vi "Deep Thought.vi"(8 "Error In":errorcluster) -> (0 "Error Out":errorcluster)   [LabVIEW 2019, in "Deep Thought.lvlib"]
doc: "Simple string based state machine."
uses:
  Deep Thought.lvlib
  <vilib>/ErrorRing/Error Ring.xnode
  Communication/Queues/MHL/MHL.lvlib
  Communication/Notifiers/Sequencer/Sequencer Handshake.lvlib
  <vilib>/Utility/error.llb/Error Cluster From Error Code.vi
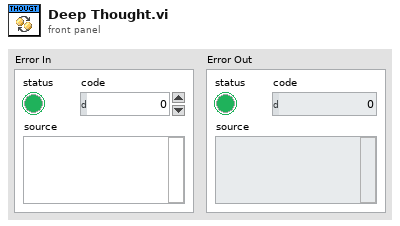
[diagram p1: front panel]
types:
  T1 = enum16{"Obtain", "Send", "Get Notifier", "Release"}
  T2 = enum16{"Obtain", "Enqueue", "Get Queue", "Flush", "Release"}
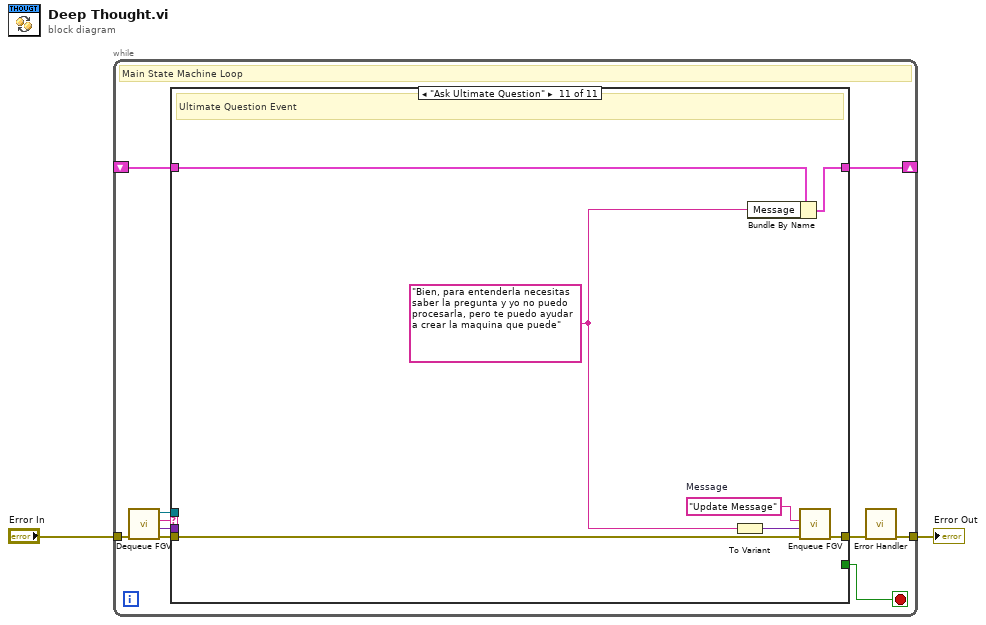
[diagram p0: block diagram]
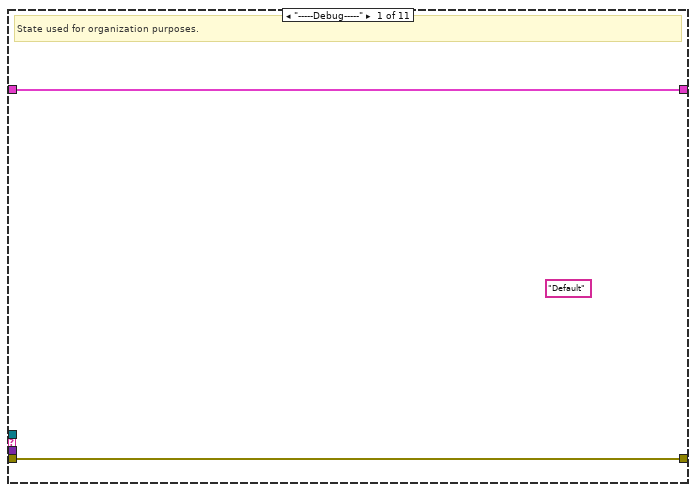
[diagram p2: hidden frame]
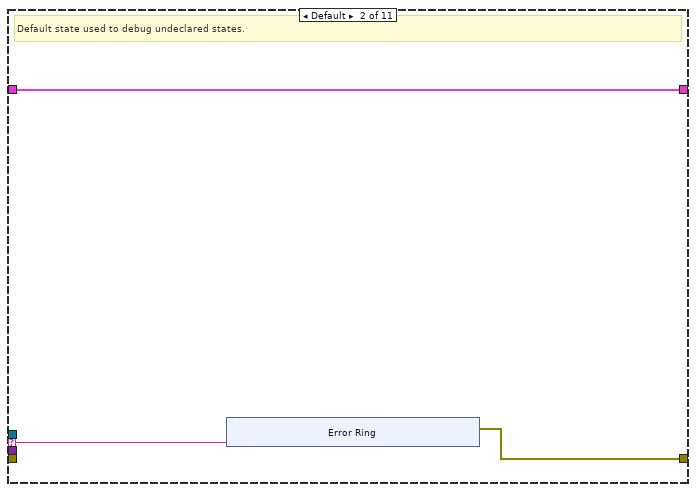
[diagram p3: hidden frame]
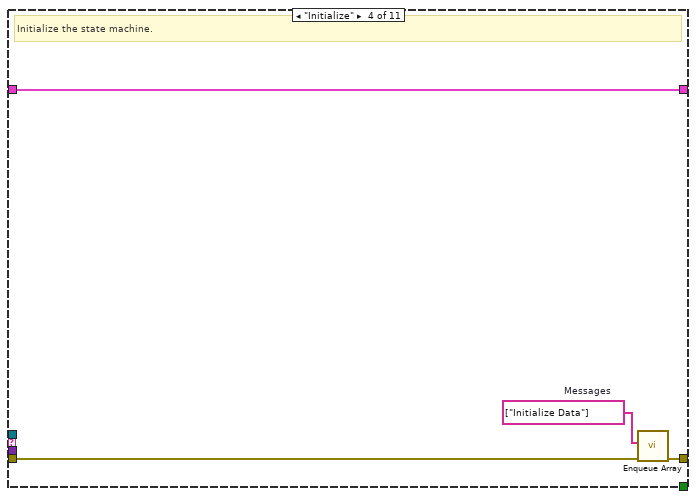
[diagram p5: hidden frame]
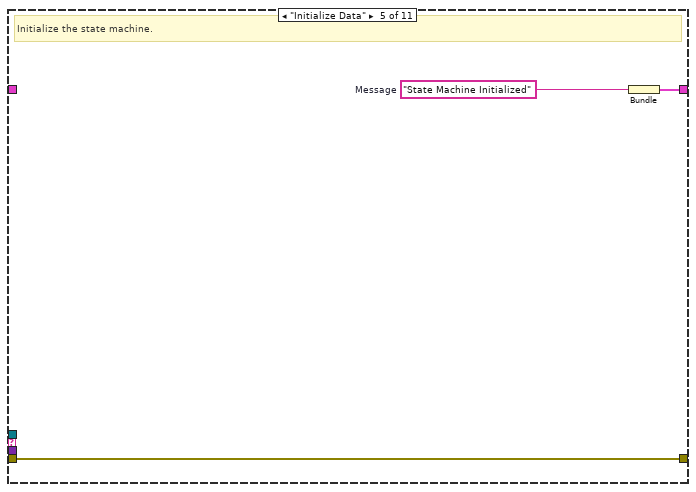
[diagram p6: hidden frame]
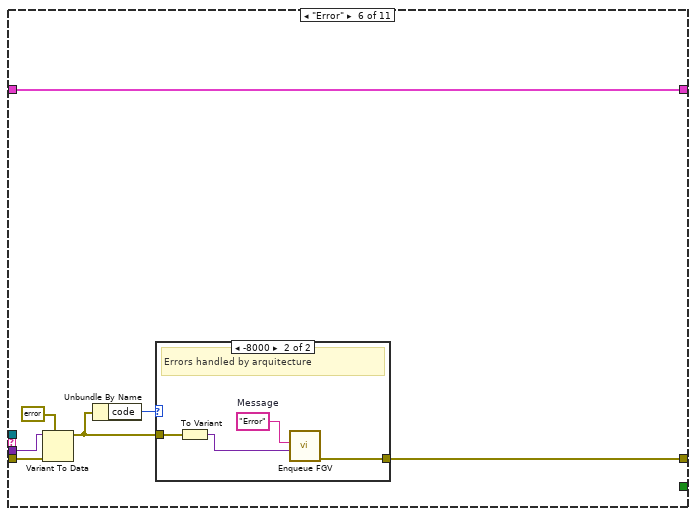
[diagram p7: hidden frame]
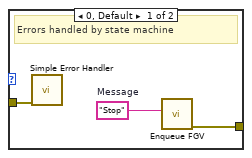
[diagram p8: hidden frame]
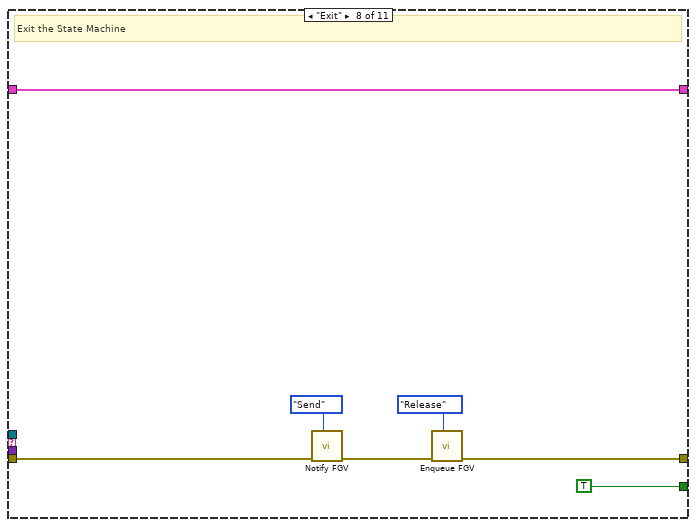
[diagram p10: hidden frame]
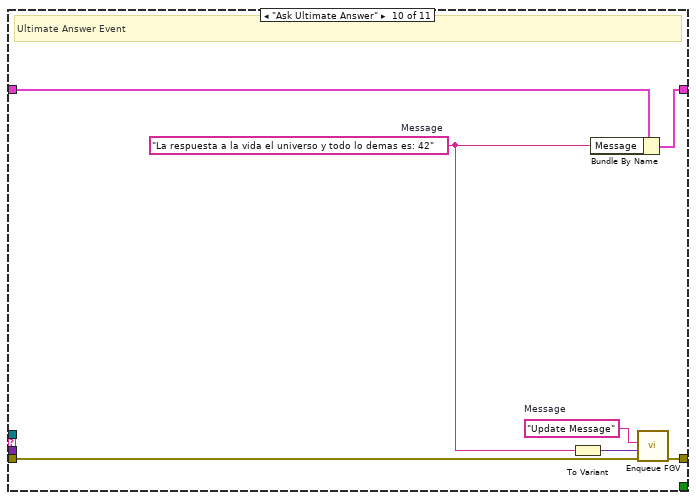
[diagram p12: hidden frame]
diagram:
  n1 = while {
    shift-right: [w11] -> _
    shift-left: _ -> [w12]
    tunnel: "Error In" -> [w9]
    tunnel: [w7] -> w2
    stop <- w10 stop-if-true
    # "Main State Machine Loop"
    n2 = call "Dequeue FGV.vi"("error in"=w9) -> ("error out"=w8:errorcluster, "Message Data"=w4:variant, "Message"=w5:string, "queue out"=w3:refnum<queue>)  [unwired: 7 in]
    n3 = case shown="\"Ask Ultimate Question\"" w5 {
      selector: w5 -> [_ w16 _ _ _ _ _ _ _ _ _]
      tunnel: w8 -> [w14 _ w26 w29 w31 w39 w48 w51 w58 w62 w67]
      tunnel: [w14 w15 w26 w30 w31 w36 w48 w54 w58 w63 w68] -> w6
      tunnel: [_ _ _ _ _ _ _ TRUE _ _ _] -> w10
      tunnel: w12 -> [w13 w17 w25 w27 _ w40 w49 w55 w57 w65 w72]
      tunnel: [w13 w17 w25 w27 w32 w40 w49 w55 w57 w64 w71] -> w11
      tunnel: w4 -> [_ _ _ _ _ w38 _ _ _ _ _]
      tunnel: w3 -> [_ _ _ _ _ _ _ _ _ _ _]
      frame "-----Debug-----" {
        (unwired) "Default" ("State")
        # "State used for organization purposes."
      }
      frame Default {
        # "Default state used to debug undeclared states."
        n4 = xnode "Error Ring"("parameter 0"=w16) -> ("error out"=w15:errorcluster)
      }
      frame "-----Core-----" {
        # "State used for organization purposes."
      }
      frame "Initialize" {
        w28 = string[] ["Initialize Data"]  # Messages
        # "Initialize the state machine."
        n5 = call "Enqueue Array.vi"("error in"=w29, "Messages"=w28) -> ("error out"=w30:errorcluster)  [unwired: 9 in]
      }
      frame "Initialize Data" {
        w33 = "State Machine Initialized"  # Message
        # "Initialize the state machine."
        n6 = Bundle("Message"=w33) -> (w32:cluster{"Message":string})  [unwired: 1 in]
      }
      frame "Error" {
        n7 = Variant To Data(error in=w39, type=errorcluster {"status"=FALSE, "code"=0, "source"=""} ("error constant"), Variant=w38) -> (data=w34:errorcluster)  [unwired: 1 out]
        n8 = Unbundle By Name(w34) -> ("code"=w35:i32)
        n9 = case shown="-8000" w35 {
          tunnel: [w43 w47] -> w36
          tunnel: w34 -> [w41 w45]
          frame 0, Default {
            w42 = "Stop"  # Message
            # "Errors handled by state machine"
            n10 = call <vilib>:"Simple Error Handler.vi"("error in (no error)"=w41) -> ()  [unwired: 4 in, 5 out]
            n11 = call "Enqueue FGV.vi"("Message"=w42) -> ("error out"=w43:errorcluster)  [unwired: 9 in, 1 out]
          }
          frame -8000 {
            w46 = "Error"  # Message
            # "Errors handled by arquitecture"
            n12 = To Variant(anything=w45) -> (Variant=w44:variant)
            n13 = call "Enqueue FGV.vi"("Message Data"=w44, "Message"=w46) -> ("error out"=w47:errorcluster)  [unwired: 8 in, 1 out]
          }
        }
      }
      frame "Stop" {
        # "Stop the State Machine"
      }
      frame "Exit" {
        # "Exit the State Machine"
        n14 = call "Notify FGV.vi"("Actions"=T1."Send", "error in"=w51) -> ("error out"=w52:errorcluster)  [unwired: 8 in, 1 out]
        n15 = call "Enqueue FGV.vi"("Actions"=T2."Release", "error in"=w52) -> ("error out"=w54:errorcluster)  [unwired: 8 in, 1 out]
      }
      frame "-----States-----" {
        # "State used for organization purposes."
      }
      frame "Ask Ultimate Answer" {
        w59 = "La respuesta a la vida el universo y todo lo demas es: 42"  # Message
        w61 = "Update Message"  # Message
        # "Ultimate Answer Event"
        n16 = To Variant(anything=w59) -> (Variant=w60:variant)
        n17 = Bundle By Name(cluster=w65, "Message"=w59) -> (w64:cluster{"Message":string})
        n18 = call "Enqueue FGV.vi"("error in"=w62, "Message Data"=w60, "Message"=w61) -> ("error out"=w63:errorcluster)  [unwired: 7 in, 1 out]
      }
      frame "Ask Ultimate Question" {
        w66 = "Bien, para entenderla necesitas saber la pregunta y yo no puedo procesarla, pero te puedo ayudar a crear la maquina que puede" ("Message")
        w70 = "Update Message"  # Message
        # "Ultimate Question Event"
        n19 = To Variant(anything=w66) -> (Variant=w69:variant)
        n20 = Bundle By Name(cluster=w72, "Message"=w66) -> (w71:cluster{"Message":string})
        n21 = call "Enqueue FGV.vi"("error in"=w67, "Message Data"=w69, "Message"=w70) -> ("error out"=w68:errorcluster)  [unwired: 7 in, 1 out]
      }
    }
    n22 = call "Error Handler.vi"("error in"=w6) -> ("dup error in"=w7:errorcluster)  [unwired: 9 in, 1 out]
  }
  "Error Out" <- w2
